vi "Capture Image.vi"(8 "error in (no error)":errorcluster, 9 "Exposure":dbl, 10 "String":string, 11 "Refnum in":T2) -> (0 "error out":errorcluster, 3 "Refnum out":T1)   [LabVIEW 2020]
doc: "Capture an Image."
uses:
  <vilib>/userdefined/High Color/IMAQdx.ctl
  <vilib>/vision/Image Controls.llb/IMAQ Image.ctl
  <vilib>/vision/driver/NI_Vision_Acquisition_Software.lvlib
  <resource>/objmgr/imaqdx.rc
panel:
  out "Image":T1(plugin-control)
  in  "error in (no error) 2":errorcluster
  in  "Exposure 2":u32
  out "error out 2":errorcluster
  in  "String 2":string
  out "Refnum out 2":T1
  in  "Refnum in 2":T2
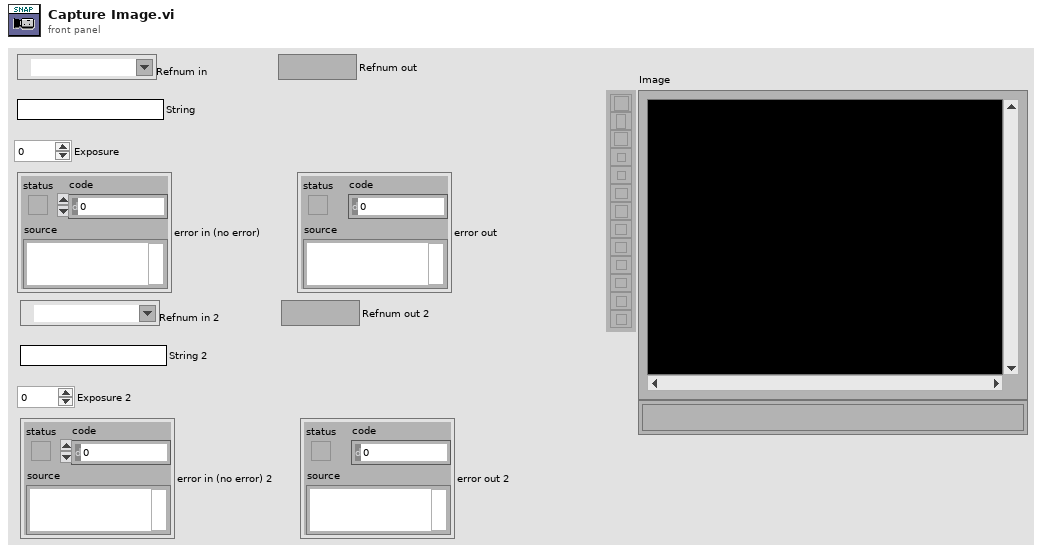
[diagram p1: front panel]
types:
  T1 = typedef "IMAQ Image.ctl" = refnum<image>
  T2 = typedef "IMAQdx.ctl" = refnum<k21>
  T3 = typedef "Image Type" = u32
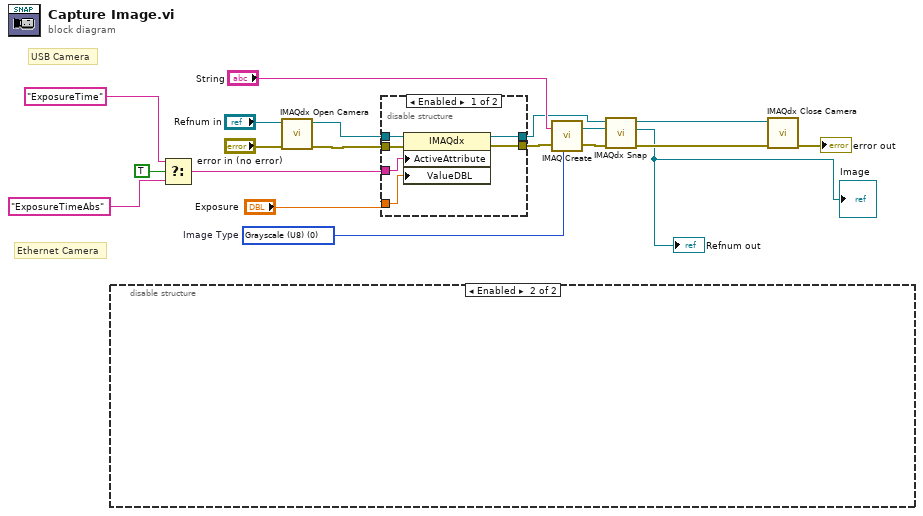
[diagram p0: block diagram]
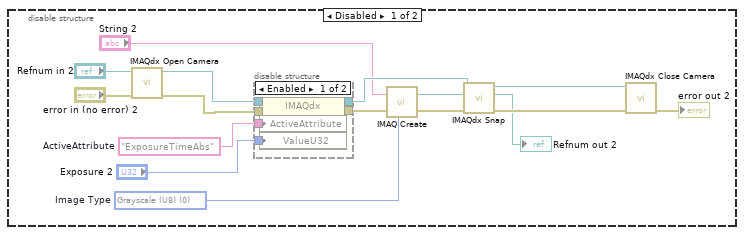
[diagram p2: hidden frame]
diagram:
  w17 = T3 0 items=["Grayscale (U8)", "Grayscale (I16)", "Grayscale (SGL)", "Complex (CSG)", "RGB (U32)", "HSL (U32)", "RGB (U64)", "Grayscale (U16)"]  # Image Type
  # "Ethernet Camera"
  # "USB Camera"
  n1 = disable-structure shown="Enabled" {
    frame Disabled {
      w23 = T3 0 items=["Grayscale (U8)", "Grayscale (I16)", "Grayscale (SGL)", "Complex (CSG)", "RGB (U32)", "HSL (U32)", "RGB (U64)", "Grayscale (U16)"]  # Image Type
      w35 = "ExposureTimeAbs"  # ActiveAttribute
      n2 = call <vilib>:"IMAQdx Open Camera.vi"("error in"="error in (no error) 2", "Session In"="Refnum in 2") -> ("error out"=w34:errorcluster, "Session Out"=w27:T2)  [unwired: 1 in, 7 out]
      n3 = disable-structure shown="Enabled" {
        disable-tunnel: [w41 w43] -> w24
        disable-tunnel: w35 -> [w40 _]
        disable-tunnel: w27 -> [w39 w42]
        disable-tunnel: "Exposure 2" -> [w38 _]
        disable-tunnel: [w37 w42] -> w30
        disable-tunnel: w34 -> [w36 w43]
        frame Enabled {
          n4 = property class="IMAQdx"(reference=w39, error in=w36, "ActiveAttribute"=w40, "ValueU32"=w38) -> (reference out=w37:T2, error out=w41:errorcluster)
        }
        frame Disabled {
        }
      }
      n5 = call "IMAQ Create"("Image Name"="String 2", "Image Type"=w23, "error in (no error)"=w24) -> ("New Image"=w21:T1, "error out"=w22:errorcluster)  [unwired: 1 in, 1 out]
      n6 = call <vilib>:"IMAQdx Snap.vi"("error in"=w22, "Image In"=w21, "Session In"=w30) -> ("error out"=w31:errorcluster, "Image Out"=→"Refnum out 2":T1, "Session Out"=w32:T2)  [unwired: 6 out]
      n7 = call <vilib>:"IMAQdx Close Camera.vi"("error in"=w31, "Session In"=w32) -> ("error out"=→"error out 2":errorcluster)  [unwired: 9 out]
    }
    frame Enabled {
    }
  }
  n8 = Select(t="ExposureTime" ("ActiveAttribute"), s=TRUE, f="ExposureTimeAbs" ("ActiveAttribute")) -> (s? t:f=w3:string)
  n9 = call <vilib>:"IMAQdx Open Camera.vi"("error in"="error in (no error)", "Session In"="Refnum in") -> ("error out"=w8:errorcluster, "Session Out"=w5:T2)  [unwired: 1 in, 7 out]
  n10 = disable-structure shown="Enabled" {
    disable-tunnel: [w49 w51] -> w16
    disable-tunnel: w5 -> [w48 w50]
    disable-tunnel: [w47 w50] -> w12
    disable-tunnel: w8 -> [w46 w51]
    disable-tunnel: w3 -> [w45 _]
    disable-tunnel: "Exposure" -> [w44 _]
    frame Enabled {
      n11 = property class="IMAQdx"(reference=w48, error in=w46, "ActiveAttribute"=w45, "ValueDBL"=w44) -> (reference out=w47:T2, error out=w49:errorcluster)
    }
    frame Disabled {
    }
  }
  n12 = call "IMAQ Create"("Image Name"="String", "Image Type"=w17, "error in (no error)"=w16) -> ("New Image"=w19:T1, "error out"=w18:errorcluster)  [unwired: 1 in, 1 out]
  n13 = call <vilib>:"IMAQdx Snap.vi"("error in"=w18, "Image In"=w19, "Session In"=w12) -> ("error out"=w11:errorcluster, "Image Out"=→"Refnum out" →"Image":T1, "Session Out"=w10:T2)  [unwired: 6 out]
  n14 = call <vilib>:"IMAQdx Close Camera.vi"("error in"=w11, "Session In"=w10) -> ("error out"=→"error out":errorcluster)  [unwired: 9 out]
